vi "Execute Open Message Handler.vi"(6 "Mouse Position":T1, 8 "User VI Ref":refnum<vi>, 9 "Menu Item Tag Suffix":string, 10 "Remaining Items":refnum<vi>[](array[refnum]), 11 "Affected Items":T2) -> (0 "Fail transaction?":bool)   [LabVIEW 2020]
doc: "This VI is part of a plug-in for modifying the LabVIEW shortcut menus. This is the execute VI which is called when the shortcut menu is chosen by the user. It performs the action of the selected menu item."
uses:
  Open Message Handler.ctl
  <vilib>/Utility/miscctls.llb/LVPositionTypeDef.ctl
panel:
  # "All controls on this panel except \"Affected Items\" have been locked to prevent accidental edits. Changing the control names or types, other than the elements of the \"Affected Items\" cluster will make the VI unusable as a menu plugin.\n\nSee Context Help for each control for details about its use."
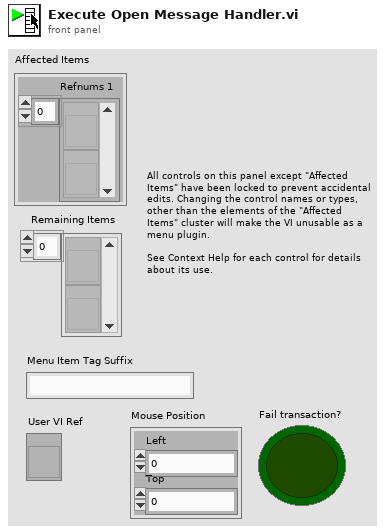
[diagram p1: front panel]
types:
  T1 = typedef "LVPositionTypeDef.ctl" = cluster{"Left":i32, "Top":i32}
  T2 = typedef "Open Message Handler.ctl" = cluster{"Refnums 1":refnum<vi>[]}
  T3 = enum8{"No dynamic dispatch VIs", "Include nearest implementation", "Include all overrides"}
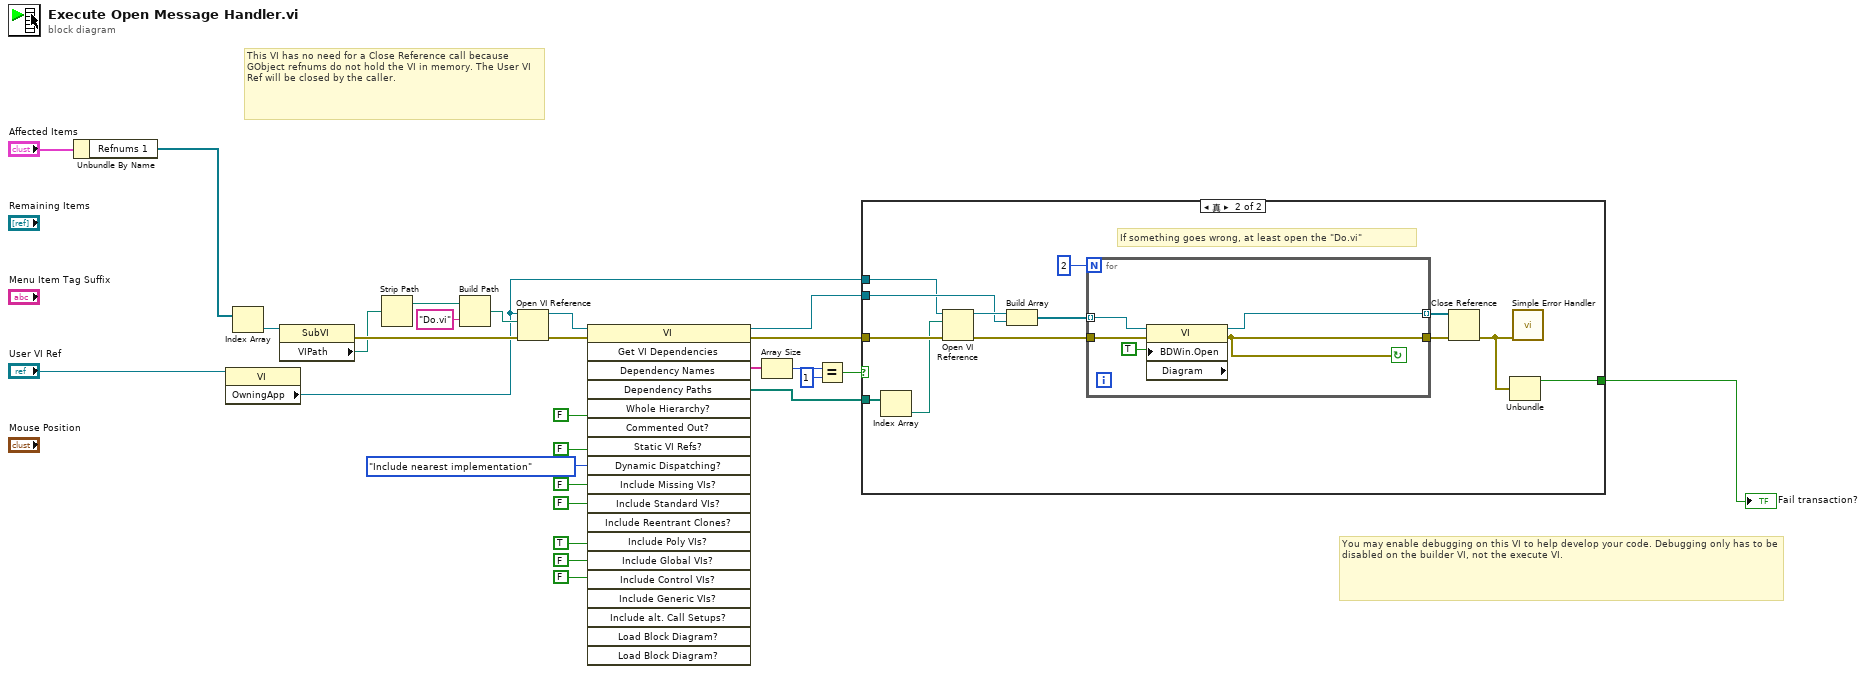
[diagram p0: block diagram]
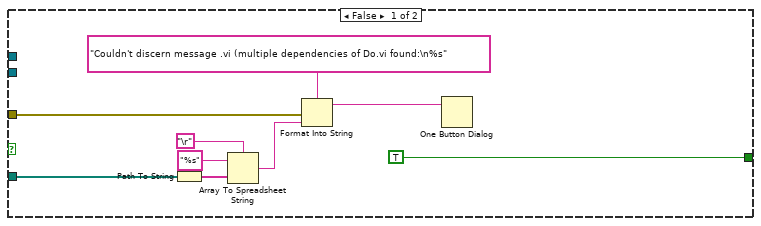
[diagram p2: hidden frame]
diagram:
  # "You may enable debugging on this VI to help develop your code. Debugging only has to be disabled on the builder VI, not the execute VI."
  # "This VI has no need for a Close Reference call because GObject refnums do not hold the VI in memory. The User VI Ref will be closed by the caller."
  n1 = Unbundle By Name("Affected Items") -> ("Refnums 1"=w3:refnum<vi>[])
  n2 = property class="VI"(reference="User VI Ref") -> ("OwningApp"=w4:refnum<vi>)  [unwired: 1 in, 2 out]
  n3 = Index Array(array=w3) -> (element=w5:refnum<vi>)  [unwired: 1 in]
  n4 = property class="SubVI"(reference=w5) -> (error out=w27:errorcluster, "VIPath"=w23:path)  [unwired: 1 in, 1 out]
  n5 = Strip Path(path=w23) -> (stripped path=w26:path)  [unwired: 1 out]
  n6 = Build Path(base path=w26, name or relative path="Do.vi") -> (appended path=w24:path)
  n7 = Open VI Reference(application reference (local)=w4, vi path=w24, error in (no error)=w27) -> (vi reference=w14:refnum<vi>, error out=w13:errorcluster)  [unwired: 3 in]
  n8 = invoke class="VI" method="Get VI Dependencies"(reference=w14, error in=w13, "Whole Hierarchy?"=FALSE, "Static VI Refs?"=FALSE, "Dynamic Dispatching?"=T3."Include nearest implementation", "Include Missing VIs?"=FALSE ("Include Missing Items?"), "Include Standard VIs?"=FALSE, "Include Poly VIs?"=TRUE, "Include Global VIs?"=FALSE, "Include Control VIs?"=FALSE) -> (reference out=w6:refnum<vi>, error out=w9:errorcluster, "Dependency Names"=w12:string[], "Dependency Paths"=w7:path[])  [unwired: 9 in, 15 out]
  n9 = Array Size(array=w12) -> (size(s)=w11:i32)
  n10 = Equal?(x=w11, y=1) -> (x = y?=w8:bool)
  n11 = case shown="真" w8 {
    tunnel: w9 -> [w31 w49]
    tunnel: w7 -> [w37 w48]
    tunnel: [TRUE ("Fail transaction?") w40] -> w1
    tunnel: w6 -> [_ w43]
    tunnel: w4 -> [_ w38]
    frame False {
      n12 = Path To String(path=w37) -> (string=w36:string[])
      n13 = Array To Spreadsheet String(delimiter (Tab)="\r", array=w36, 3:"%s" ("format string")) -> (spreadsheet string=w32:string)
      n14 = Format Into String(format string="Couldn't discern message .vi (multiple dependencies of Do.vi found:\n%s", error in=w31, w32) -> (resulting string=w30:string)  [unwired: 1 in, 1 out]
      n15 = One Button Dialog(message=w30) -> ()  [unwired: 1 in, 1 out]
    }
    frame True {
      # "If something goes wrong, at least open the \"Do.vi\""
      n16 = Index Array(array=w48) -> (element=w47:path)  [unwired: 1 in]
      n17 = Open VI Reference(application reference (local)=w38, vi path=w47, error in (no error)=w49) -> (vi reference=w44:refnum<vi>, error out=w50:errorcluster)  [unwired: 3 in]
      n18 = Build Array(w44, w43) -> (w42:refnum<vi>[])
      n19 = for {
        N: 2 -> [_]
        tunnel: w42 -> [w52] mode=indexing
        tunnel: [w51] -> w41 mode=indexing
        tunnel: w50 -> [w53]
        tunnel: [w55] -> w46
        stop <- w55 continue-if-true
        n20 = property class="VI" props=["BDWin.Open", "Diagram"](reference=w52, error in=w53, "BDWin.Open"=TRUE ("Block Diagram Window:Open")) -> (reference out=w51:refnum<vi>, error out=w55:errorcluster)  [unwired: 1 out]
      }
      n21 = Close Reference(reference=w41, error in (no error)=w46) -> (error out=w39:errorcluster)
      n22 = Unbundle(w39) -> ("status"=w40:bool)  [unwired: 2 out]
      n23 = call <vilib>:"Simple Error Handler.vi"("error in (no error)"=w39) -> ()  [unwired: 4 in, 5 out]
    }
  }
  "Fail transaction?" <- w1
